vi "GetSimpleBatteryState.vi"() -> ()   [LabVIEW 2021]
uses:
  Enums/BatteryHealth_Enum.ctl
panel:
  in  "unloaded voltage":dbl
  out "BatteryHealth":T1
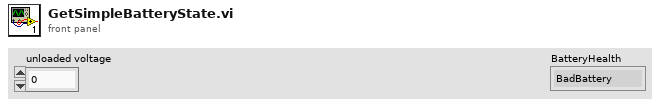
[diagram p1: front panel]
types:
  T1 = typedef "BatteryHealth_Enum.ctl" = enum16{"BadBattery", "GoodBattery"}
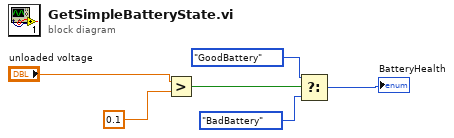
[diagram p0: block diagram]
diagram:
  n1 = Greater?(x="unloaded voltage", y=0.1) -> (0:w3:bool)
  n2 = Select(t=BatteryHealth_Enum."GoodBattery" ("BatteryState 2"), s=w3, f=BatteryHealth_Enum."BadBattery" ("BatteryState 2")) -> (s? t:f=→"BatteryHealth":T1)
